vi "Concatinate MODBUS regs (SubVI).vi"(9 "LSB reg num":u16, 11 "registers array in":u16[](array[numeric])) -> (1 "register data":i32, 3 "registers array out":u16[](array[numeric]))   [LabVIEW 2015]
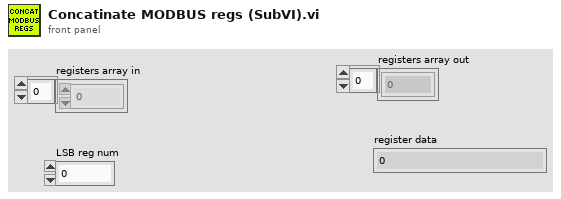
[diagram p1: front panel]
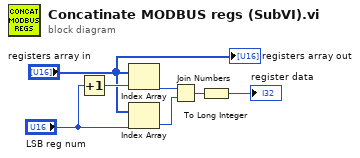
[diagram p0: block diagram]
diagram:
  n1 = Increment(x="LSB reg num") -> (x+1=w4:u16)
  n2 = Index Array(array="registers array in", index=w4) -> (element=w7:u16)
  n3 = Index Array(array="registers array in", index="LSB reg num") -> (element=w6:u16)
  n4 = Join Numbers(hi=w7, lo=w6) -> ((hi.lo)=w3:u32)
  n5 = To Long Integer(number=w3) -> (32bit integer=→"register data":i32)
  "registers array out" <- "registers array in"
